vi "LabVIEW.vi"() -> ()   [LabVIEW 2022 SP3]
uses:
  Program Files/National Instruments/LabVIEW 2022/examples/Instrument IO/Serial/support/Serial - XON-XOFF Characters.ctl
  Program Files/National Instruments/LabVIEW 2022/examples/Instrument IO/Serial/support/Serial - ASCII Characters.ctl
  Program Files/National Instruments/LabVIEW 2022/examples/Instrument IO/Serial/support/Serial - Settings.ctl
  <vilib>/Instr/_visa.llb/VISA Configure Serial Port (Instr).vi
  <vilib>/addons/control/pid/pid.llb/PID (DBL).vi
  <vilib>/addons/control/pid/NI_PID_pid.lvlib
panel:
  out "Real height m":dbl
  in  "Tab Control":enum32{"Manual", "PID"}(tab)
  in  "Pump flow":dbl(slide)=5.0 scale=0.0..24.0
  in  "PID gains":T1={"proportional gain (Kc)"=1.0, "integral time (Ti, min)"=0.01, "derivative time (Td, min)"=0.0} {"derivative time (Td, min)" format="%.12f"; "integral time (Ti, min)" format="%.6f"; "proportional gain (Kc)" format="%.3f"}
  in  "setpoint":dbl=10.0 format="%#_13g"
  out "output":dbl=3.773309999999965 format="%.2f"
  out "Plant Output":dbl=24.999997972053873 format="%.2f"
  in  "Flow Gain":dbl=25.5 format="%#_13g"
  out "PWM Value":u8=96
  in  "AI1_Ofset":dbl=50.0
  in  "AI1_Gain":dbl=-0.2 format="%#_13g"
  in  "AI0_Ofset":dbl=50.0
  in  "AI0_Gain":dbl=-0.25 format="%#_13g"
  out "AI1":i32=511
  out "AI0":i32=418
  in  "VISA resource name":refnum<visa-resource-name>="COM4"
  out "Waveform Chart":dbl[][](graph)=[[24.999997972053873, 9.957040000000006, -52.0]]
  in  "Simullation parameters":T2={"static gain"=2.5, "lag (s)"=2.5, "deadtime (s)"=0.001, "load"=0.0, "deadband"=0.0, "sensor noise"=0.0, "initial PV"=0.2, "plant noise"=0.0} {"plant noise" format="%.2f"; "initial PV" format="%.2f"; "sensor noise" format="%.2f"; "lag (s)" format="%.2f"; "deadtime (s)" format="%.2f"; "deadband" format="%.1f"; "load" format="%.2f"; "static gain" format="%.8f"}
  in  "dt (s)":dbl=0.3 format="%.3f"
  in  "output saturation range":cluster{"output high":dbl, "output low":dbl}={"output high"=inf, "output low"=-inf}
  in  "stop":bool
  # "Aquisition Parameters"
  # "Control parameters"
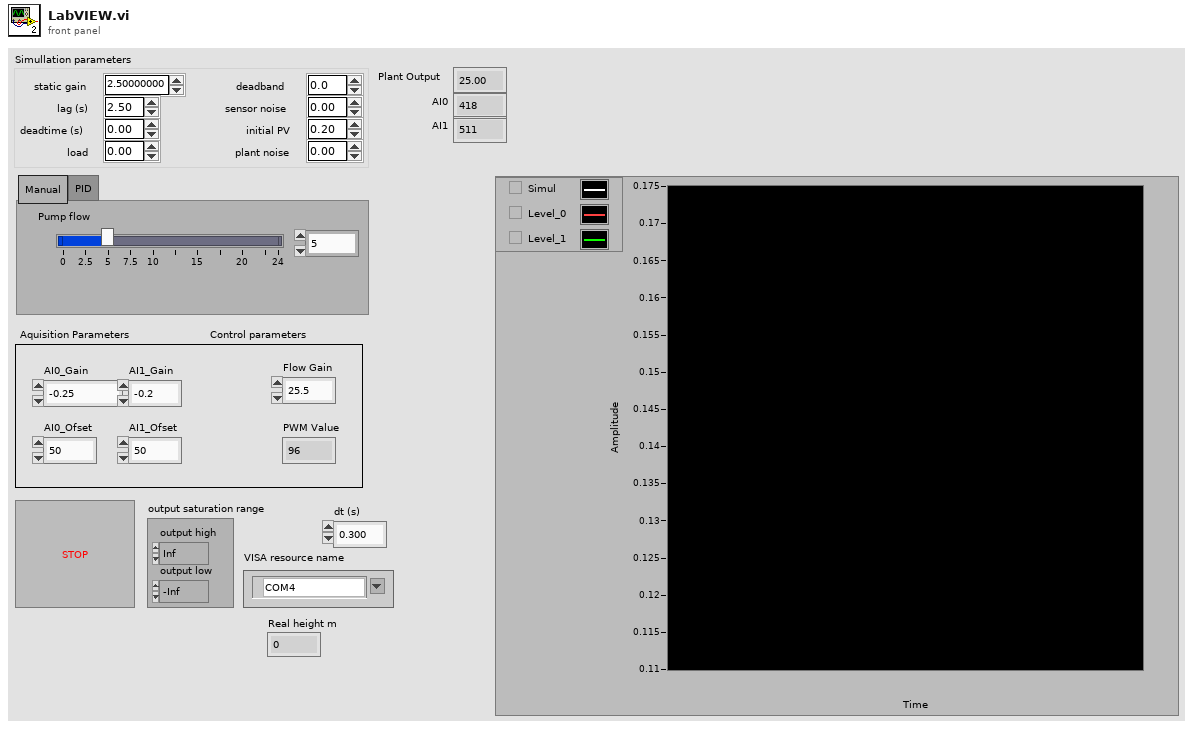
[diagram p1: front panel]
types:
  T1 = cluster{"proportional gain (Kc)":dbl, "integral time (Ti, min)":dbl, "derivative time (Td, min)":dbl}
  T2 = cluster{"static gain":dbl, "lag (s)":dbl, "deadtime (s)":dbl, "load":dbl, "deadband":dbl, "sensor noise":dbl, "initial PV":dbl, "plant noise":dbl}
  T3 = typedef "Serial - Settings.ctl" = cluster{"baud rate":u32, "data bits":u16, "parity":enum16{"None", "Odd", "Even", "Mark", "Space"}, "stop bits":u16, "flow control":u16}
  T4 = typedef "Serial - XON-XOFF Characters.ctl" = cluster{"XON":T5, "XOFF":T5}
  T5 = typedef "Serial - ASCII Characters.ctl" = enum16{"NUL", "SOH", "STX", "ETX", "EOT", "ENQ", "ACK", "BEL", "BS", "HT", "LF", "VT", "FF", "CR", "SO", "SI", "DLE", "DC1", "DC2", "DC3", "DC4", "NAK", "SYN", "ETB", "CAN", "EM", "SUB", "ESC", "FS", "GS", "RS", "US", "SP", "!", "\"", "#", "$", "%", "&", "'", "(", ")", "*", "+", ",", "- (-)", ".", "/", "0", "1", "2", "3", "4", "5", "6", "7", "8", "9", ":", ";", "<", "=", ">", "?", "@", "A", "B", "C", "D", "E", "F", "G", "H", "I", "J", "K", "L", "M", "N", "O", "P", "Q", "R", "S", "T", "U", "V", "W", "X", "Y", "Z", "[", "\\", "]", "^", "_", "`", "a", "b", "c", "d", "e", "f", "g", "h", "i", "j", "k", "l", "m", "n", "o", "p", "q", "r", "s", "t", "u", "v", "w", "x", "y", "z", "{", "|", "}", "~"}
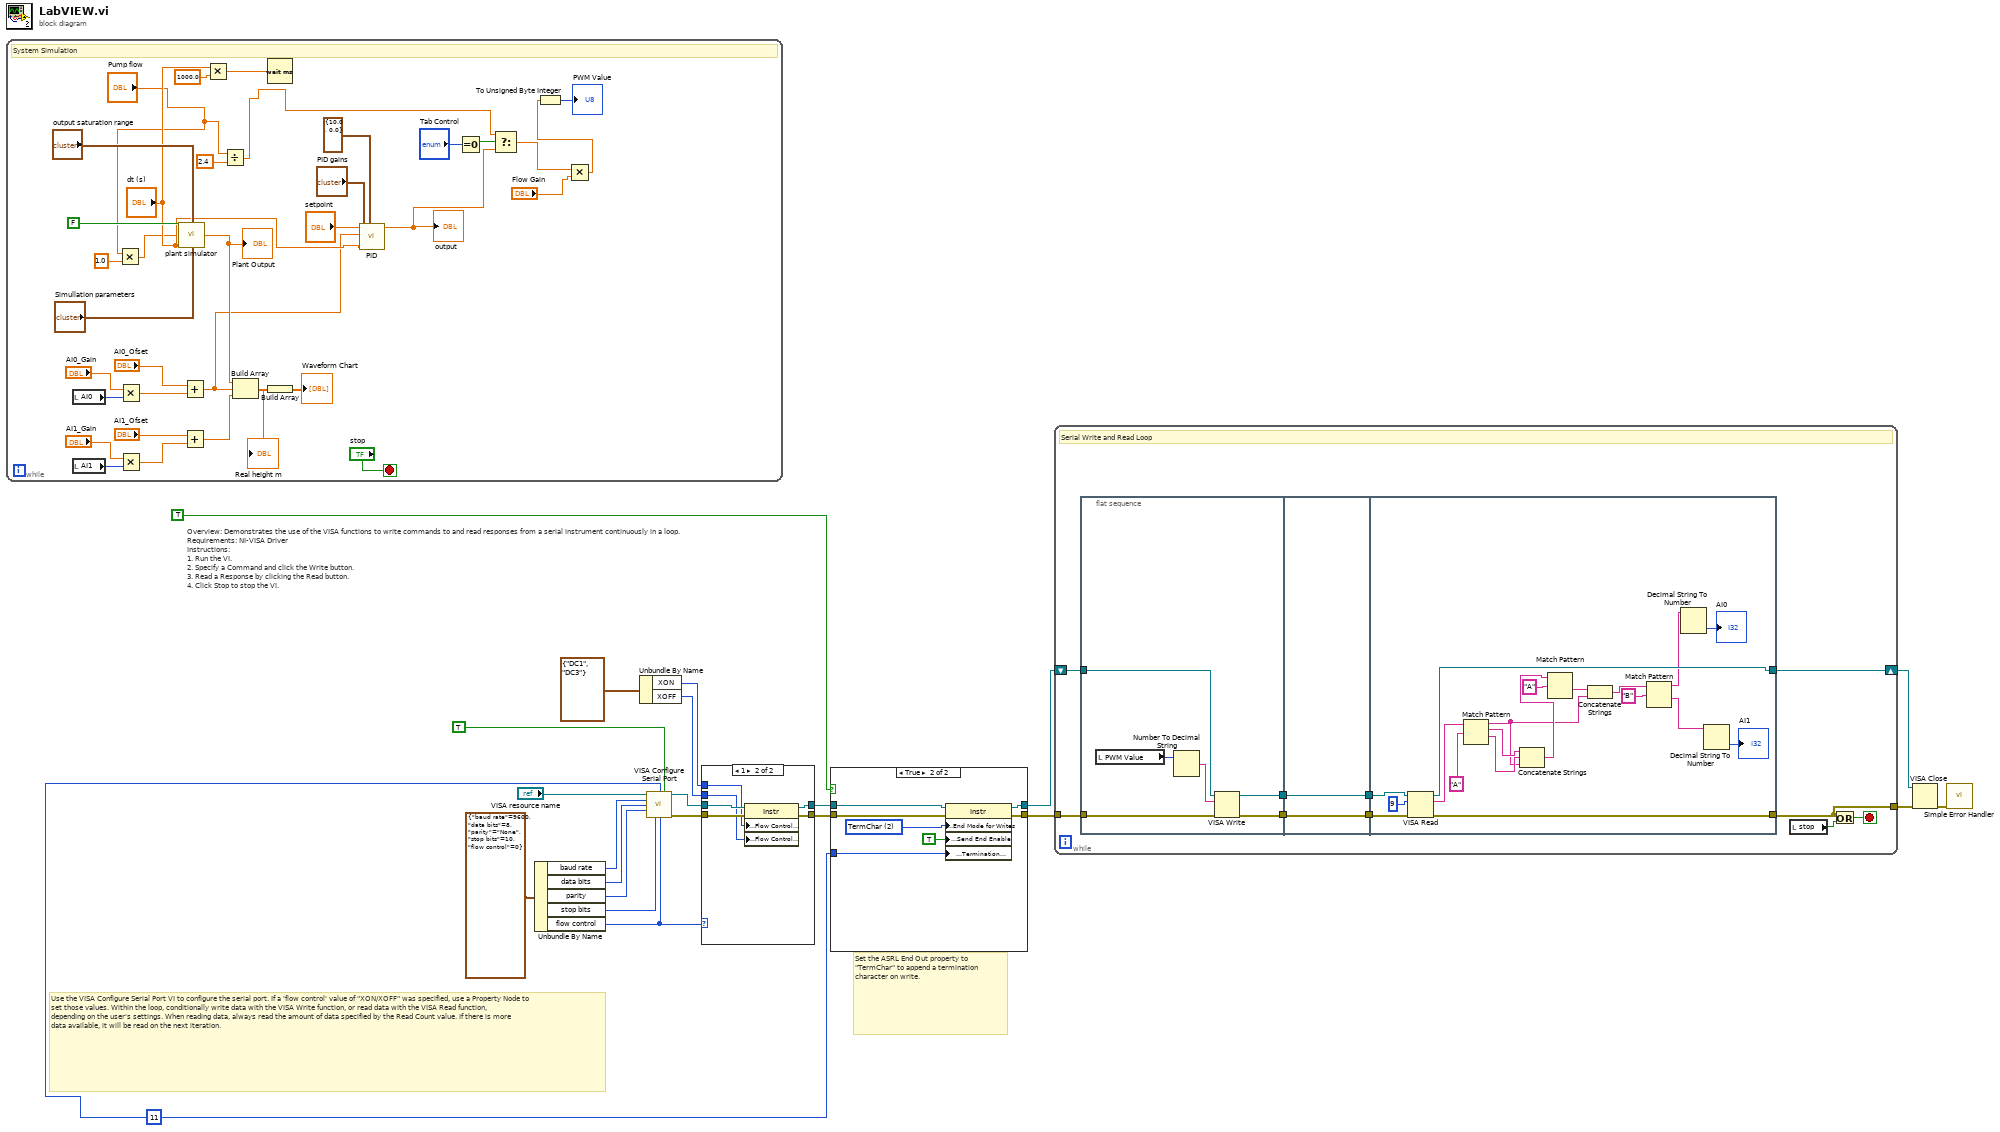
[diagram p0: block diagram]
diagram:
  w1 = u8 11 ("Termination Character")
  # "Set the ASRL End Out property to \"TermChar\" to append a termination character on write."
  # "Use the VISA Configure Serial Port VI to configure the serial port. If a 'flow control' value of \"XON/XOFF\" was specified, use a Property Node to set those values. Within the loop, conditionally write data with the VISA Write function, or read data with the VISA Read function, depending on the user's settings. When reading data, always read the amount of data specified by the Read Count value. If there is more data available, it will be read on the next iteration."
  # "Overview: Demonstrates the use of the VISA functions to write commands to and read responses from a serial instrument continuously in a loop.\nRequirements: NI-VISA Driver\nInstructions:\n1. Run the VI.\n2. Specify a Command and click the Write button.\n3. Read a Response by clicking the Read button.\n4. Click Stop to stop the VI."
  n1 = while {
    stop <- "stop" stop-if-true
    # "System Simulation"
    n2 = local read "AI0"() -> (w37:i32)
    n3 = local read "AI1"() -> (w43:i32)
    n4 = Multiply(x="Pump flow", y=1.0) -> (x*y=w26:dbl)
    n5 = Multiply(x="AI0_Gain", y=w37) -> (x*y=w50:dbl)
    n6 = Multiply(x="AI1_Gain", y=w43) -> (x*y=w47:dbl)
    n7 = call "plant simulator.vi"("output saturation range"="output saturation range", "Plant Input"=w26, "dt (s)"="dt (s)", "reinitialize? (F)"=FALSE, "Simullation parameters"="Simullation parameters") -> ("Plant Output"=w45:dbl)  [unwired: 10 in]
    "Plant Output" <- w45
    n8 = Add(x="AI0_Ofset", y=w50) -> (x+y=w33:dbl)
    "Real height m" <- w33
    n9 = Add(x="AI1_Ofset", y=w47) -> (x+y=w44:dbl)
    n10 = Multiply(x="dt (s)", y=1000.0) -> (x*y=w52:dbl)
    n11 = Divide(x="Pump flow", y=2.4) -> (x/y=w23:dbl)
    n12 = Build Array(w45, w33, w44) -> (w42:dbl[])
    n13 = Wait (ms)(milliseconds to wait=w52) -> ()  [unwired: 1 out]
    n14 = Build Array(w42) -> (→"Waveform Chart":dbl[][])
    n15 = call-poly <vilib>:"PID.vi"("output range"=cluster{"output high":dbl, "output low":dbl} {"output high"=10.0, "output low"=0.0}, "dt (s)"="dt (s)", "PID gains"="PID gains", "process variable"=w33, "setpoint"="setpoint") -> ("output"=w30:dbl)  [unwired: 5 in, 1 out]
    "output" <- w30
    n16 = Equal To 0?(x="Tab Control") -> (x = 0?=w31:bool)
    n17 = Select(t=w23, s=w31, f=w30) -> (s? t:f=w28:dbl)
    n18 = Multiply(x=w28, y="Flow Gain") -> (x*y=w29:dbl)
    n19 = To Unsigned Byte Integer(number=w29) -> (unsigned 8bit integer=→"PWM Value":u8)
  }
  n20 = Unbundle By Name(T3 {"baud rate"=9600, "data bits"=8, "parity"=enum."None", "stop bits"=10, "flow control"=0} ("Serial Settings")) -> ("baud rate"=w15:u32, "data bits"=w16:u16, "parity"=w17:enum16{"None", "Odd", "Even", "Mark", "Space"}, "stop bits"=w18:u16, "flow control"=w9:u16)
  n21 = Unbundle By Name(T4 {"XON"=enum."DC1", "XOFF"=enum."DC3"} ("XON/XOFF Characters")) -> ("XON"=w8:T5, "XOFF"=w7:T5)
  n22 = call-poly "VISA Configure Serial Port"("VISA resource name"="VISA resource name", "termination char\n(0xA = '\\n' = LF)"=w1, "Enable Termination\nChar (T)"=TRUE ("End Read on Termination Character?"), "baud rate (9600)"=w15, "data bits (8)"=w16, "parity (0:none)"=w17, "stop bits (10: 1 bit)"=w18, "flow control (0:none)"=w9) -> ("VISA resource name out"=w19:refnum<visa-resource-name>, "error out"=w20:errorcluster)  [unwired: 2 in, 4 out]
  n23 = case shown="1" w9 {
    tunnel: [w58 w65] -> w6
    tunnel: [w59 w64] -> w4
    tunnel: w20 -> [w58 w63]
    tunnel: w19 -> [w59 w62]
    tunnel: w8 -> [_ w61]
    tunnel: w7 -> [_ w60]
    frame Default {
    }
    frame 1 {
      n24 = property class="Instr"(reference=w62, error in=w63, "Serial Settings:Flow Control XON Character"=w61, "Serial Settings:Flow Control XOFF Character"=w60) -> (reference out=w64:refnum<visa-resource-name>, error out=w65:errorcluster)
    }
  }
  n25 = case shown="True" TRUE ("End Write on Termination Character?") {
    tunnel: w4 -> [w66 w74]
    tunnel: w6 -> [w67 w73]
    tunnel: [w66 w72] -> w3
    tunnel: [w67 w71] -> w5
    tunnel: w1 -> [_ w69]
    frame False {
    }
    frame True {
      w70 = u16 2 items=["None", "LastBit", "TermChar", "Break"] ("Serial Settings:Serial End Mode for Writes")
      n26 = property class="Instr"(reference=w74, error in=w73, "Serial Settings:End Mode for Writes"=w70, "Message Based Settings:Send End Enable"=TRUE, "Message Based Settings:Termination Character"=w69) -> (reference out=w72:refnum<visa-resource-name>, error out=w71:errorcluster)
    }
  }
  n27 = while {
    shift-right: [w84] -> w10
    shift-left: w3 -> [w75]
    tunnel: w5 -> [w76]
    tunnel: [w82] -> w11
    stop <- w83 stop-if-true
    # "Serial Write and Read Loop"
    n28 = flat-sequence {
      tunnel: [w86] -> w78
      tunnel: [w87] -> w77
      tunnel: w76 -> [w89]
      tunnel: w75 -> [w88]
      tunnel: [w92] -> w80
      tunnel: [w91] -> w79
      tunnel: w78 -> [w92]
      tunnel: w77 -> [w91]
      tunnel: [w111] -> w84
      tunnel: [w108] -> w82
      tunnel: w80 -> [w110]
      tunnel: w79 -> [w109]
      frame #0 {
        n29 = local read "PWM Value"() -> (w90:u8)
        n30 = Number To Decimal String(number=w90) -> (decimal integer string=w85:string)  [unwired: 1 in]
        n31 = VISA Write(VISA resource name=w88, write buffer=w85, error in (no error)=w89) -> (VISA resource name out=w86:refnum<visa-resource-name>, error out=w87:errorcluster)  [unwired: 1 out]
      }
      frame #1 {
      }
      frame #2 {
        n32 = VISA Read(VISA resource name=w110, byte count=u32 9 ("Read Count"), error in (no error)=w109) -> (VISA resource name out=w111:refnum<visa-resource-name>, read buffer=w93:string, error out=w108:errorcluster)  [unwired: 1 out]
        n33 = Match Pattern(string=w93, regular expression="A") -> (before substring=w96:string, match substring=w98:string, after substring=w97:string)  [unwired: 1 in, 1 out]
        n34 = Concatenate Strings(w98, w97, w96) -> (w99:string)
        n35 = Match Pattern(string=w99, regular expression="A") -> (after substring=w102:string)  [unwired: 1 in, 3 out]
        n36 = Concatenate Strings(w102, w96) -> (w101:string)
        n37 = Match Pattern(string=w101, regular expression="B") -> (before substring=w95:string, after substring=w94:string)  [unwired: 1 in, 2 out]
        n38 = Decimal String To Number(string=w95) -> (number=→"AI0":i32)  [unwired: 2 in, 1 out]
        n39 = Decimal String To Number(string=w94) -> (number=→"AI1":i32)  [unwired: 2 in, 1 out]
      }
    }
    n40 = local read "stop"() -> (w81:bool)
    n41 = Or(x=w82, y=w81) -> (x .or. y?=w83:bool)
  }
  n42 = VISA Close(VISA resource name=w10, error in (no error)=w11) -> (error out=w12:errorcluster)
  n43 = call <vilib>:"Simple Error Handler.vi"("error in (no error)"=w12) -> ()  [unwired: 1 in, 8 out]
